vi "MecaWheelPos_New.vi"(8 "RearRightPosition":dbl format="%19.3f", 9 "RearLeftPosition":dbl format="%19.3f", 10 "FrontRightPosition":dbl format="%19.3f", 11 "FrontLeftPosition":dbl format="%19.3f") -> (3 "MECA_WHEEL_POSITIONS":T1 {"RearRight" format="%19.3f"; "RearLeft" format="%19.3f"; "FrontRight" format="%19.3f"; "FrontLeft" format="%19.3f"})   [LabVIEW 2019, in "Trajectory_Library.lvlib"]
doc: "Constructs a MecanumDriveWheelPosition data structure.\n\nParameters:\n - Left Front Position - Distance measured by left front wheel (meters)\n - Right Front Position - Distance measured by right front wheel (meters)\n - Left Rear Position - Distance measured by left rear wheel (meters)\n - Right Rear Position - Distance measured by right rear wheel (meters)\n\nReturns:\n - Meca_wheel_Position- Data structure"
uses:
  Trajectory_Library.lvlib
  TypeDef/MECA_WHEEL_POSITIONS.ctl
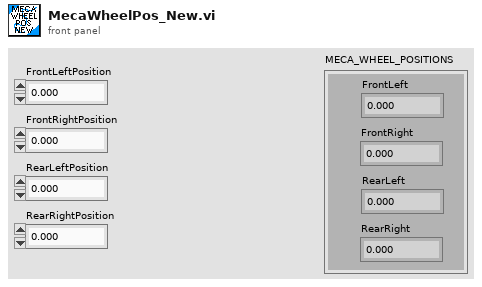
[diagram p1: front panel]
types:
  T1 = typedef "Trajectory_Library.lvlib/MECA_WHEEL_POSITIONS.ctl" = cluster{"FrontLeft":dbl, "FrontRight":dbl, "RearLeft":dbl, "RearRight":dbl}
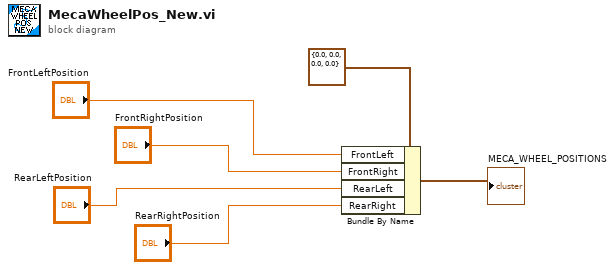
[diagram p0: block diagram]
diagram:
  n1 = Bundle By Name(cluster=T1 {"FrontLeft"=0.0, "FrontRight"=0.0, "RearLeft"=0.0, "RearRight"=0.0} ("MECA_WHEEL_POSITIONS"), "FrontLeft"="FrontLeftPosition", "FrontRight"="FrontRightPosition", "RearLeft"="RearLeftPosition", "RearRight"="RearRightPosition") -> (→"MECA_WHEEL_POSITIONS":T1)
